vi "GFITS_SeZcntProgress.vi"(8 "error in (no error)":errorcluster, 10 "counter":i32, 11 "Database RefNum":T1) -> (0 "error out":errorcluster)   [LabVIEW 2016]
uses:
  DBSHAND/private/vis/DatabaseHand_RefNum.ctl
  DBSHAND/private/vis/DatabaseHand_Element_Set(I32).vi
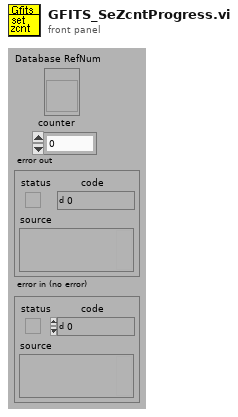
[diagram p1: front panel]
types:
  T1 = typedef "DatabaseHand_RefNum.ctl" = refnum<vi>
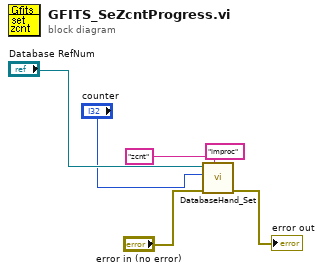
[diagram p0: block diagram]
diagram:
  (unwired) "improc" ("group")
  n1 = call-poly "DatabaseHand_Set.vi"("name"="zcnt" ("value"), "error in (no error)"="error in (no error)", "value"="counter", "Database RefNum in"="Database RefNum") -> ("error out"=→"error out":errorcluster)  [unwired: 4 in, 3 out]
